vi "IR Transmit Raw.vi"(0 "Arduino Resource":T2={"VISA resource"="", "Board Type"=enum."Uno", "Connection Type"=enum."USB / Serial", "Bytes Per Packet (15)"=15}, 5 "IR Type":T1, 7 "Data":u32, 9 "Number Of Bits (32 Max)":u8=32, 11 "Error In":errorcluster) -> (4 "Arduino Resource":T2={"VISA resource"="", "Board Type"=enum."Uno", "Connection Type"=enum."USB / Serial", "Bytes Per Packet (15)"=15}, 15 "Error Out":errorcluster)   [LabVIEW 2011, in "LabVIEW Interface for Arduino.lvlib"]
uses:
  <vilib>/LabVIEW Interface for Arduino/LabVIEW Interface for Arduino.lvlib
  <vilib>/LabVIEW Interface for Arduino/Private/Type Defs/Arduino Resource.ctl
  <vilib>/LabVIEW Interface for Arduino/Private/Type Defs/Board Type.ctl
  <vilib>/LabVIEW Interface for Arduino/Private/Type Defs/IR Type.ctl
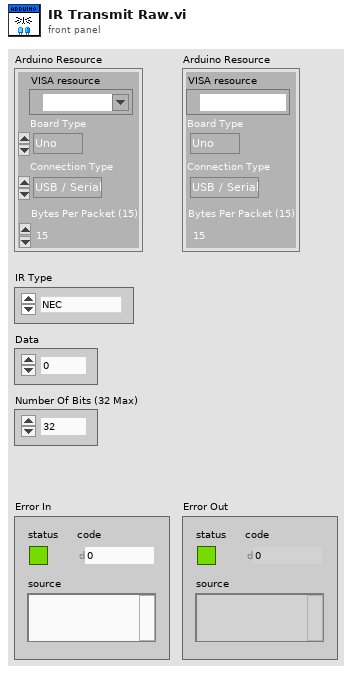
[diagram p1: front panel]
types:
  T1 = typedef "LabVIEW Interface for Arduino.lvlib/IR Type.ctl" = enum8{"NEC", "Sony", "RC5", "RC6"}
  T2 = typedef "LabVIEW Interface for Arduino.lvlib/Arduino Resource.ctl" = cluster{"VISA resource":refnum<visa-resource-name>, "Board Type":T3, "Connection Type":enum8{"USB / Serial"}, "Bytes Per Packet (15)":u8}
  T3 = typedef "LabVIEW Interface for Arduino.lvlib/Board Type.ctl" = enum16{"Uno", "Dimuelanove w/Atmega 328", "Mega 2560"}
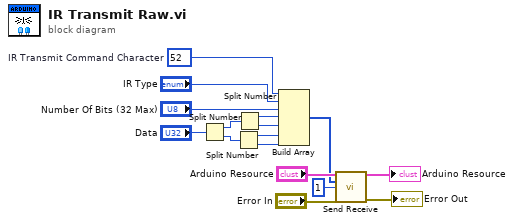
[diagram p0: block diagram]
diagram:
  w9 = u8 52  # IR Transmit Command Character
  n1 = Split Number(x="Data") -> (hi(x)=w5:u16, lo(x)=w6:u16)
  n2 = Split Number(x=w6) -> (hi(x)=w2:u8, lo(x)=w1:u8)
  n3 = Split Number(x=w5) -> (hi(x)=w4:u8, lo(x)=w3:u8)
  n4 = Build Array(w9, "IR Type", "Number Of Bits (32 Max)", w4, w3, w2, w1) -> (w12:u8[])
  n5 = call <vilib>:"Send Receive.vi"("Arduino Resource"="Arduino Resource", "Data"=w12, "Bytes To Read (0)"=u32 1, "error in"="Error In") -> ("Arduino Resource"=→"Arduino Resource":T2, "error out"=→"Error Out":errorcluster)  [unwired: 9 in, 1 out]
